vi "SPOL_LabVIEW_Variables.vi"() -> (3 "Variables":dbl[](array[numeric]) format="%.3g")   [LabVIEW 2009]
doc: "Reads the SPOL_LabVIEW_Variables input file\nSig Gen Frequency"
uses:
  <vilib>/regexp/Match Regular Expression.xnode
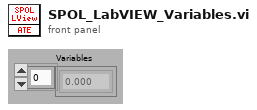
[diagram p1: front panel]
types:
  T1 = enum16{"open", "replace", "create", "open or create", "replace or create", "replace or create with confirmation"}
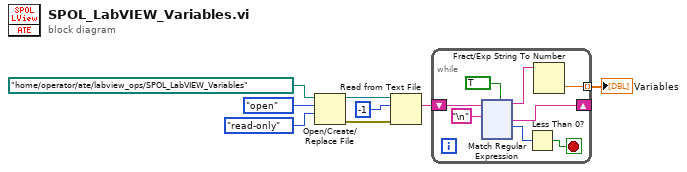
[diagram p0: block diagram]
diagram:
  n1 = Open/Create/Replace File(file path (use dialog)=path "/home/operator/ate/labview_ops/SPOL_LabVIEW_Variables", operation (0:open)=T1."open", access (0:read/write)=enum16{"read/write", "read-only", "write-only"}."read-only") -> (refnum out=w5:refnum<file>, error out=w3:errorcluster)  [unwired: 3 in, 1 out]
  n2 = Read from Text File(file (use dialog)=w5, count=-1, error in=w3) -> (text=w2:string)  [unwired: 1 in, 3 out]
  n3 = while {
    shift-right: [w13] -> _
    shift-left: w2 -> [w16]
    tunnel: [w10] -> w1 mode=indexing
    stop <- w9 stop-if-true
    n4 = xnode "Match Regular Expression"("input string"=w16, "regular expression"="\n", "multiline? (F)"=TRUE) -> ("before match"=w11:string, "after match"=w13:string, "offset past match"=w12:i32)  [unwired: 3 in, 2 out]
    n5 = Less Than 0?(x=w12) -> (x < 0?=w9:bool)
    n6 = Fract/Exp String To Number(string=w11) -> (number=w10:dbl)  [unwired: 3 in, 1 out]
  }
  "Variables" <- w1
